vi "Disable Heating.vi"(8 "error in (no error)":errorcluster, 10 "Start Time":timestamp, 11 "Thermal Chamber Response Simlator In":refnum<class "Thermal Chamber Response Simlator.lvclass">) -> (0 "error out":errorcluster, 3 "Thermal Chamber Response Simlator Out":refnum<class "Thermal Chamber Response Simlator.lvclass">)   [LabVIEW 2020, in "Thermal Chamber Response Simlator.lvclass"]
uses:
  Thermal Chamber Response Simlator.lvclass
  Thermal Chamber Response Simlator.lvclass/Thermal Chamber Response Simlator.ctl
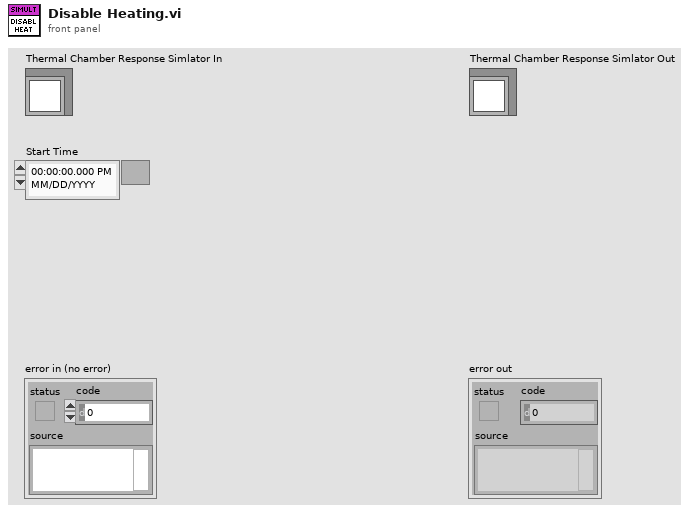
[diagram p1: front panel]
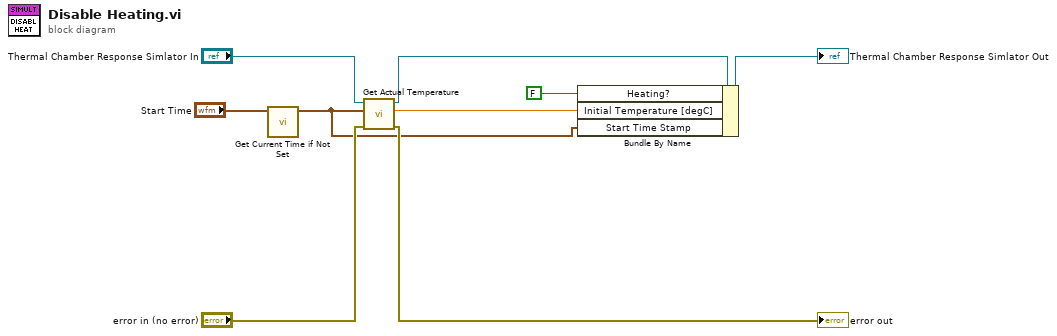
[diagram p0: block diagram]
diagram:
  n1 = call "Get Current Time if Not Set.vi"("Start Time"="Start Time") -> ("seconds since 1Jan1904"=w1:timestamp)  [unwired: 10 in]
  n2 = call "Get Actual Temperature.vi"("error in (no error)"="error in (no error)", "Time Stamp"=w1, "Thermal Chamber Response Simlator In"="Thermal Chamber Response Simlator In") -> ("error out"=→"error out":errorcluster, "Actual Temperature [degC]"=w6:dbl, "Thermal Chamber Response Simlator Out"=w4:refnum<class "Thermal Chamber Response Simlator.lvclass">)  [unwired: 6 in]
  n3 = Bundle By Name(cluster=w4, "Heating?"=FALSE, "Initial Temperature [degC]"=w6, "Start Time Stamp"=w1) -> (→"Thermal Chamber Response Simlator Out":refnum<class "Thermal Chamber Response Simlator.lvclass">)
